vi "Control Refs Wrapper.vi"   [LabVIEW 2015]
uses:
  <vilib>/LV-Control-Refs/LV-Control-Refs.xnode
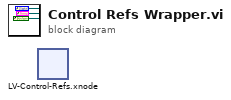
[diagram p0: block diagram]
diagram:
  n1 = xnode "LV-Control-Refs.xnode"() -> ()  [unwired: 1 in, 2 out]
